vi "MotionGlobals.vi"() -> ()   [LabVIEW 2022 SP3]
uses:
  -ScanSystem/Controls/location.ctl
  -ScanSystem/Controls/EKG_Mode.ctl
  -ScanSystem/Controls/ScanType2.ctl
  -ScanSystem/Controls/Breath_Mode.ctl
  Spectrometers/OceanOptics/OceanOpticsVIs.llb/SpectrometerType.ctl
  NI_controller/-NI_MotionRoutines/MotionParameters.ctl
  NI_controller/-NI_MotionRoutines/MotionSys.ctl
  ScanAxis.ctl
  3rdAxis.ctl
  Misc Programs/VideoCardEnum/VideoCard.ctl
panel:
  in  "Limit Warned?":bool
  in  "Preview Configed?":bool
  in  "Debug Mode?":bool
  in  "NVIDIA Card":T1
  in  "Vz Counter":i16
  in  "2D Counter":i16
  in  "Overview Counter":i16
  in  "Scanning Speed Multiplier":dbl=1.0
  in  "USB Gate Per Sample":bool
  in  "c mm/mics":sgl=1.5
  in  "Root Save Path":path=path "G:/Data/2019-09-16"
  in  "Motion Settings":T2={"No Motion?"=FALSE, "Motion System"=enum."NI 735x", "Motion Bd ID"=1, "Motion Profile"="SMAC1", "# Axis"=1, "Reverse Z axis?"=TRUE, "SMAC Axis"=0, "scan pair"=enum."x-(y) scan", "RT fps"=6.0, "Steps per mm"=[1000, 1000, 1000, 1000], "Motor Parameters"={"velocity ct/s"=[10000.0, 10000.0, 10000.0, 50000.0], "accel ct/s^2"=[50000.0, 50000.0, 50000.0, 200000.0]}, "One Way Scan"=FALSE, "Reverse One Way Scan"=FALSE, "Global Position (mm)"=[], "Plane"=0, "Distance between\nscan lines (um)"=100.0, "Distance between\nscan planes (um)"=100.0, "number of scan planes"=1, "Total steps in line"=0, "Xtra plane\ndistance  (um)"=100, "Xtra planes "=1, "Add Axis"=FALSE, "overshoot cts"=200, "BKPT Shift"=0, "Scan Start Time (ms)"=0, "ESP VISA"="GPIB::1::INSTR", "3rd Axis"=1, "GL Ref Out"=refnum, "Galil Address"=""} {"3rd Axis" items=["x", "y", "z", "w"]; "Xtra planes" min=1; "Xtra plane\ndistance  (um)" min=0; "Distance between\nscan planes (um)" format="%.2f"; "Distance between\nscan lines (um)" format="%.2f"; "SMAC Axis" items=["None"=0, "Axis 1"=1, "Axis 2"=2, "Axis 3"=3, "Axis 4"=4, "Axis 5"=5, "Axis 6"=6, "Axis 7"=7, "Axis 8"=8, "Vector Space 1"=17, "Vector Space 2"=18, "Vector Space 3"=19, "Vector Space 4"=20]; "Motion Bd ID" min=1 max=32 step=1}
  out "Ocean Wrapper":u32
  in  "Main Spectrometer":T6 items=["No Spectrometer", "Ocean QE_Pro"]
  in  "Filter Prams":T7={"low cutoff"=5, "order"=81, "high cutoff"=65}
  in  "Dopp Gate?":bool
  in  "Resp Wait (ms)":u32=400
  in  "Save Temp":bool
  in  "CTR PRF?":bool
  in  "FlipFlop Source":refnum<k21>="Dev1 FlipFlop"
  in  "Multi Trig#":i32=1 min=1
  in  "SavePath":path=path "G:/Data/2019-09-16"
  out "5CH Pulser Tasks":refnum<k21>[](array[refnum])
  in  "Breath Divide":i32
  in  "NI Switch":refnum<k15>
  in  "DAQ Range":cluster{"Max V":dbl, "Min V":dbl}={"Max V"=1.0, "Min V"=-1.0} {"Max V" format="%0.2f"; "Min V" format="%0.2f"}
  in  "Breath Trig":T8 items=["Respir Trig Off", "Respir Ring1 (Ch1)", "Respir Ch0", "Dig Edge"]
  in  "Done":i32
  in  "Save&Read Time":i32
  in  "Acq Time (ms)":i32
  in  "Type of scan":T9=enum."M Scan With Therapy Burst"
  in  "Multi Trig?":bool
  out "Compression Parameters":T10 {"Tukey taper" min=50 max=1000 format="%.2f"; "F2 (MHz)" format="%.3f"; "F1 (MHz)" format="%.3f"}
  in  "EKG Gate?":T11 items=["Retro/Prosp Off", "Prosp Ext EKG", "Prosp IQ EKG", "Retro EKG", "Retro IQ", "Retro No EKG"]
  out "DAQmx Task 1":refnum<k21>
  out "DAQmx Task 0":refnum<k21>
  in  "TempPath":path=path "G:/DataBuffer"
  in  "Location":T12=enum."WCM Main"
  in  "33250(T)/33120(F)":bool=TRUE
  in  "No GPIB?":bool
  # "Microscopy Scaning Counters"
  # "task IDs"
  # "Acq Modes"
  # "1-D and 2-D B scan settings"
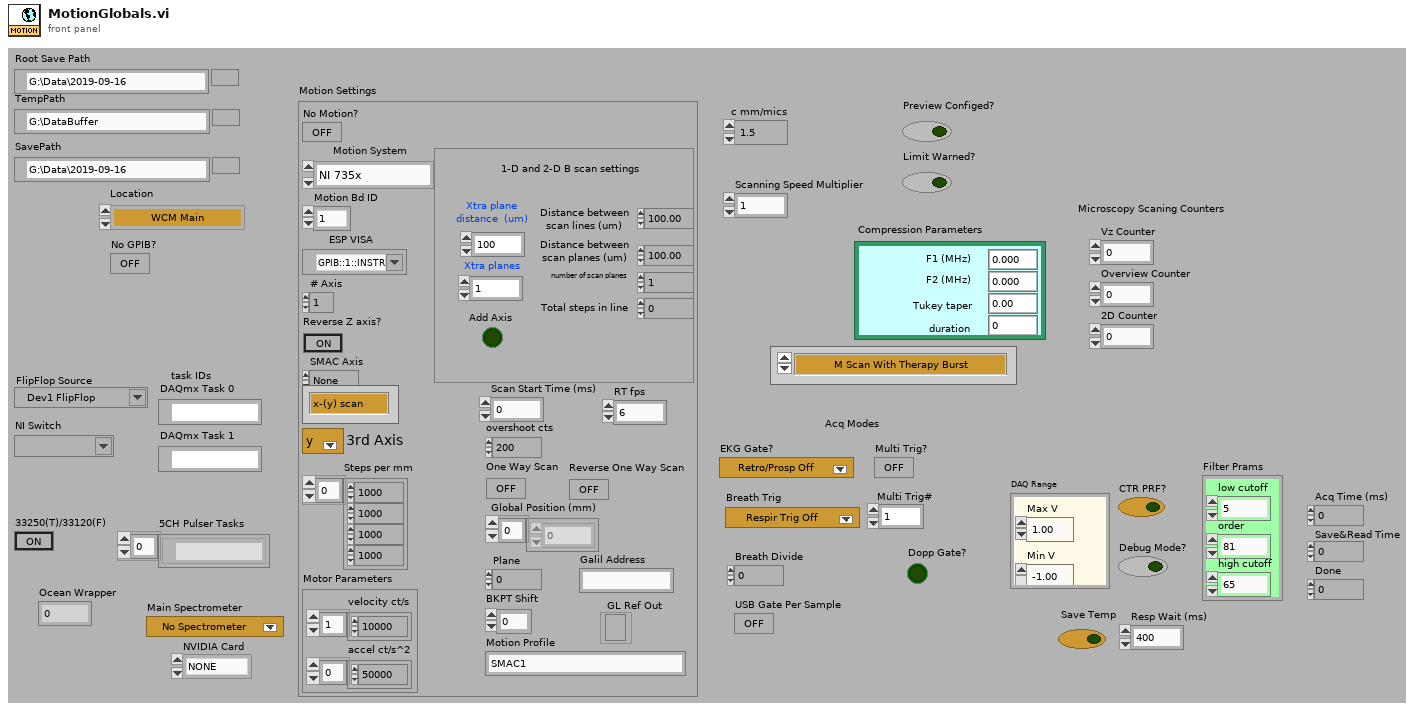
[diagram p1: front panel]
types:
  T1 = typedef "VideoCard.ctl" = enum16{"NONE", "UNKNOWN", "k620", "FX 3800", "GTX 970", "P1000"}
  T2 = typedef "MotionParameters.ctl" = cluster{"No Motion?":bool, "Motion System":T3, "Motion Bd ID":u8, "Motion Profile":string, "# Axis":i8, "Reverse Z axis?":bool, "SMAC Axis":u16, "scan pair":T4, "RT fps":sgl, "Steps per mm":i32[], "Motor Parameters":cluster{"velocity ct/s":dbl[], "accel ct/s^2":dbl[]}, "One Way Scan":bool, "Reverse One Way Scan":bool, "Global Position (mm)":dbl[], "Plane":i32, "Distance between\nscan lines (um)":sgl, "Distance between\nscan planes (um)":sgl, "number of scan planes":i32, "Total steps in line":i32, "Xtra plane\ndistance  (um)":i32, "Xtra planes ":i32, "Add Axis":bool, "overshoot cts":i32, "BKPT Shift":i32, "Scan Start Time (ms)":u32, "ESP VISA":refnum<visa-resource-name>, "3rd Axis":T5, "GL Ref Out":refnum<k7>, "Galil Address":string}
  T3 = typedef "MotionSys.ctl" = enum16{"MM3000", "NI 735x", "Newport ESP", "No Motion Card", "Galil"}
  T4 = typedef "ScanAxis.ctl" = enum16{"y-(x) scan", "x-(y) scan", "z-(x) scan", "z-(y) scan", "y-(z) scan", "x-(z) scan", "w-(x) scan", "w-(y) scan", "w-(z) scan", "x-(w) scan", "y-(w) scan", "z-(w) scan"}
  T5 = typedef "3rdAxis.ctl" = u16
  T6 = typedef "SpectrometerType.ctl" = u16
  T7 = cluster{"low cutoff":i32, "order":i32, "high cutoff":i32}
  T8 = typedef "Breath_Mode.ctl" = u16
  T9 = typedef "ScanType2.ctl" = enum16{"Therapy With Scan", "M scan", "M Scan With Therapy Burst", "1-D B Scan", "1-D B Scan With Therapy Burst", "2-D B Scan", "2-D B Scan With Therapy Burst", "Rotational Scan", "1-D B-Scan PRF", "2-D B-Scan PRF", "Real-Time Scan", "Contrast Agents", "1-D w/ Real-Time Set Up", "Dual Transducer", "Acoustic Microscopy", "Hydrophone Scanning"}
  T10 = cluster{"F1 (MHz)":sgl, "F2 (MHz)":sgl, "Tukey taper":sgl, "duration":sgl}
  T11 = typedef "EKG_Mode.ctl" = u16
  T12 = typedef "location.ctl" = enum16{"Automatic", "WCM Main", "Hawaii", "Columbia MM3000", "Columbia  NI System", "NYU", "RRI 2", "UHI Allen", "CUMC RT", "Chiba", "Stony Brook", "WCM Microscopy", "WCM Aeoretch", "WCM Optics Lab", "WCM Main 2Axis", "WCM Rotation", "WCM SAM SMAC", "SERI GP"}
diagram:
